vi "ykgw_fgv.vi"(7 "mode":enum16{"read", "write"}(ring), 10 "error in (no error)":errorcluster, 11 "Data in":dbl[](array[numeric])) -> (1 "phase current":dbl, 2 "error out":errorcluster, 3 "Data out":dbl[](array[numeric]), 4 "DC_power":dbl, 5 "Invertor Output Power":dbl)   [LabVIEW 2019]
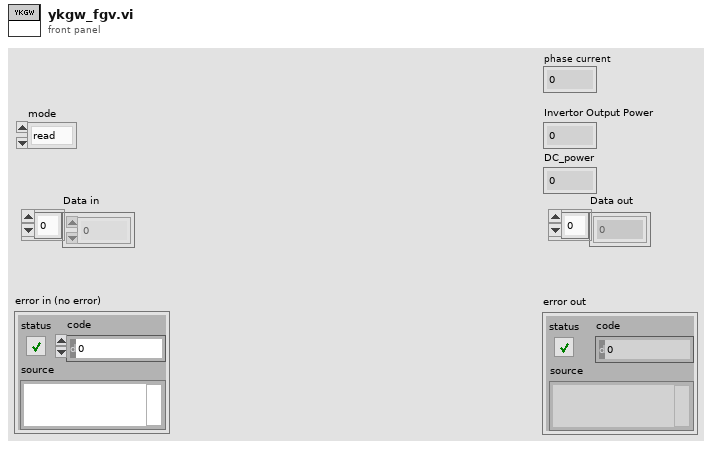
[diagram p1: front panel]
types:
  T1 = cluster{"Data in[0]":dbl, "Data in[1]":dbl, "Data in[2]":dbl, "Data in[3]":dbl, "Data in[4]":dbl, "Data in[5]":dbl, "Data in[6]":dbl, "Data in[7]":dbl, "Data in[8]":dbl}
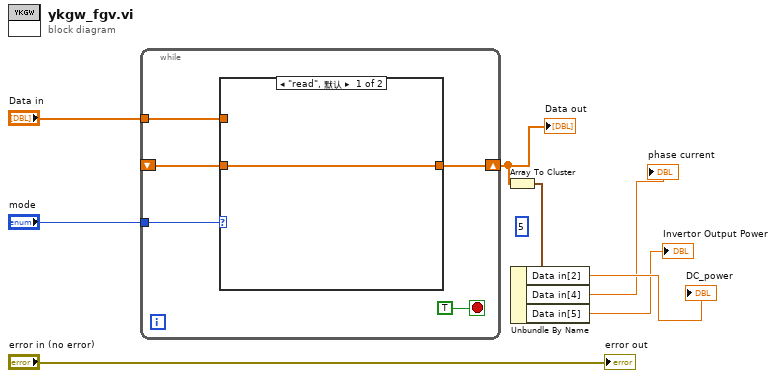
[diagram p0: block diagram]
diagram:
  (unwired) 5 ("index")
  n1 = while {
    tunnel: "mode" -> [w13]
    tunnel: "Data in" -> [w12]
    shift-right: [w11] -> w5
    shift-left: _ -> [w10]
    stop <- TRUE stop-if-true
    n2 = case shown="\"read\", 默认" w13 {
      tunnel: [w14 w15] -> w11
      tunnel: w12 -> [_ w15]
      tunnel: w10 -> [w14 _]
      frame "read", Default {
      }
      frame "write" {
      }
    }
  }
  "Data out" <- w5
  n3 = Array To Cluster(array=w5) -> (cluster=w4:T1)
  n4 = Unbundle By Name(w4) -> ("Data in[2]"=→"DC_power":dbl, "Data in[4]"=→"phase current":dbl, "Data in[5]"=→"Invertor Output Power":dbl)
  "error out" <- "error in (no error)"
